vi "Symphony Average Spectra.vi"(1 "Repetitions":i32, 2 "Raw Spectra":i32[][](array[numeric])) -> (0 "Raw Spectrum":dbl[](array[numeric]))   [LabVIEW 2010]
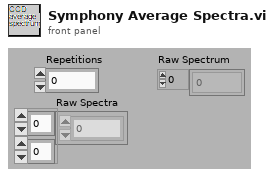
[diagram p1: front panel]
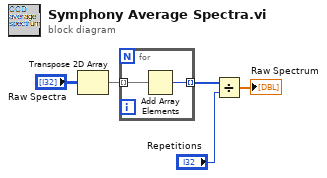
[diagram p0: block diagram]
diagram:
  n1 = Transpose 2D Array(2D array="Raw Spectra") -> (transposed array=w3:i32[][])
  n2 = for {
    tunnel: w3 -> [w7] mode=indexing
    tunnel: [w6] -> w4 mode=indexing
    n3 = Add Array Elements(numeric array=w7) -> (sum=w6:i32)
  }
  n4 = Divide(x=w4, y="Repetitions") -> (x/y=→"Raw Spectrum":dbl[])
